vi "Calculator_Calculator-setup.vi"(11 "test case ID":string) -> (1 "Numeric 2":i32=3, 2 "Numeric":i32=4)   [LabVIEW 2020]
doc: "The setup VI should be executed before the VI under test in the harness VI. In this VI you can prepare the environment and the inputs of the VI under test.\n\nSee the Help Document for more information. (<b>Help</b> > <b>InstaCoverage Help...</b>)"
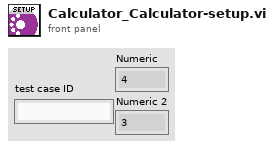
[diagram p1: front panel]
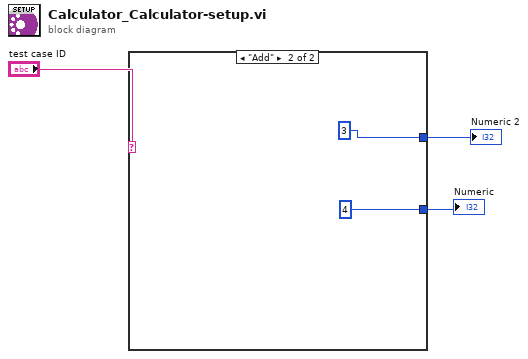
[diagram p0: block diagram]
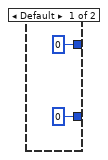
[diagram p2: hidden frame]
diagram:
  n1 = case shown="\"Add\"" "test case ID" {
    tunnel: [0 4] -> w2
    tunnel: [0 3] -> w1
    frame Default {
    }
    frame "Add" {
    }
  }
  "Numeric" <- w2
  "Numeric 2" <- w1
